vi "U3 Two 32-bit Frequency Measurements.vi"() -> ()   [LabVIEW 2021]
panel:
  out "Frequency (FIO5)":dbl format="%.2f"
  out "Period (FIO5)":dbl format="%.6f"
  out "Iteration":i32
  out "Frequency (FIO4)":dbl format="%.2f"
  out "Period (FIO4)":dbl format="%.6f"
  in  "error in":errorcluster
  in  "Address":string="1"
  in  "FirstFound":bool=TRUE
  in  "stop":bool
  out "Counter1 Diff (FIO6)":u32
  out "error out":errorcluster
  out "Error Message":string
  # "Each iteration, this VI measures the frequency on FIO4 and FIO5 using timer mode 2 (32-bit\nperiod measurement).  Also reads the count on FIO6 and\ndisplays the difference from the previous iteration, with the idea that the same signal can\nbe connected to FIO4/FIO5 and FIO6 for comparison of period timing\nversus pulse counting."
  # "seconds"
  # "seconds"
  # "This VI passes a timer\nbase clock constant that\nis valid for hardware V1.21.\nFor hardware V1.20 change\nLJ_tc48MHZ_DIV to LJ_tc24MHZ_DIV."
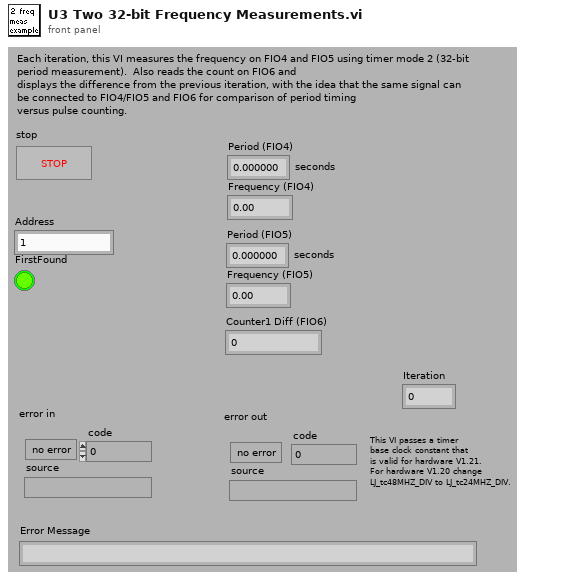
[diagram p1: front panel]
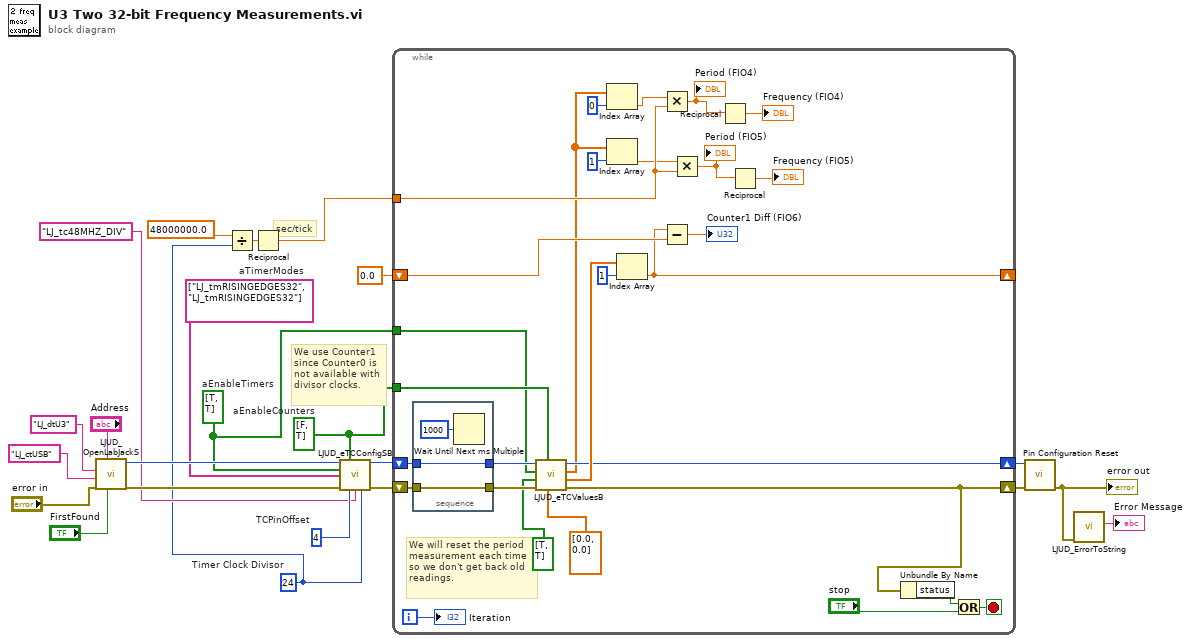
[diagram p0: block diagram]
diagram:
  w8 = 4  # TCPinOffset
  w5 = bool[] [FALSE, TRUE]  # aEnableCounters
  w4 = bool[] [TRUE, TRUE]  # aEnableTimers
  w6 = 24  # Timer Clock Divisor
  w9 = string[] ["LJ_tmRISINGEDGES32", "LJ_tmRISINGEDGES32"]  # aTimerModes
  # "We use Counter1\nsince Counter0 is\nnot available with\ndivisor clocks."
  # "sec/tick"
  n1 = call "LJUD_OpenLabJackS.vi"("FirstFound"="FirstFound", "Address"="Address", "error in"="error in", "ConnectionType"="LJ_ctUSB", "DeviceType"="LJ_dtU3") -> ("error out"=w13:errorcluster, "Handle"=w12:i32)  [unwired: 4 in, 1 out]
  n2 = Divide(x=48000000.0, y=w6) -> (x/y=w18:dbl)
  n3 = Reciprocal(x=w18) -> (1/x=w17:dbl)
  n4 = call "LJUD_eTCConfigSB.vi"("Handle In"=w12, "aEnableCounters"=w5, "aEnableTimers"=w4, "aTimerModes"=w9, "error in"=w13, "TCPinOffset"=w8, "TimerClockBase"="LJ_tc48MHZ_DIV" ("Timer Clock Base"), "TimerClockDivisor"=w6) -> ("Handle Out"=w11:i32, "error out"=w10:errorcluster)  [unwired: 6 in]
  n5 = while {
    tunnel: w4 -> [w25]
    tunnel: w5 -> [w27]
    shift-left: 0.0 ("TimerClockConfig") -> [w40]
    shift-right: [w38] -> _
    tunnel: w17 -> [w33]
    shift-left: w10 -> [w51]
    shift-right: [w31] -> w2
    shift-left: w11 -> [w52]
    shift-right: [w32] -> w3
    i -> [w37]
    stop <- w45 stop-if-true
    # "We will reset the period\nmeasurement each time\nso we don't get back old\nreadings."
    n6 = stacked-sequence {
      tunnel: [w54] -> w48
      tunnel: [w53] -> w47
      tunnel: w52 -> [w54]
      tunnel: w51 -> [w53]
      frame #0 {
        n7 = Wait Until Next ms Multiple(millisecond multiple=u32 1000) -> ()  [unwired: 1 out]
      }
    }
    n8 = call "LJUD_eTCValuesB.vi"("aTimerValues Write"=dbl[] [0.0, 0.0] ("TimerValues"), "aReadCounters"=w27, "error in"=w47, "aUpdateResetTimers"=bool[] [TRUE, TRUE] ("UpdateReset Timers"), "aReadTimers"=w25, "Handle In"=w48) -> ("error out"=w31:errorcluster, "aCounterValues"=w50:dbl[], "aTimerValues Read"=w28:dbl[], "Handle Out"=w32:i32)  [unwired: 2 in]
    n9 = Index Array(array=w28, index=0 ("Index")) -> (element=w34:dbl)
    n10 = Index Array(array=w28, index=1 ("Index")) -> (element=w30:dbl)
    n11 = Index Array(array=w50, index=1 ("Index")) -> (element=w38:dbl)
    n12 = Multiply(x=w34, y=w33) -> (x*y=w42:dbl)
    "Period (FIO4)" <- w42
    n13 = Subtract(x=w38, y=w40) -> (x-y=→"Counter1 Diff (FIO6)":dbl)
    n14 = Multiply(x=w30, y=w33) -> (x*y=w36:dbl)
    "Period (FIO5)" <- w36
    n15 = Reciprocal(x=w42) -> (1/x=→"Frequency (FIO4)":dbl)
    n16 = Reciprocal(x=w36) -> (1/x=→"Frequency (FIO5)":dbl)
    n17 = Unbundle By Name(w31) -> ("status"=w44:bool)
    n18 = Or(x=w44, y="stop") -> (x .or. y?=w45:bool)
    "Iteration" <- w37
  }
  n19 = call "Pin Configuration Reset.vi"("error in"=w2, "Handle In"=w3) -> ("error out"=w1:errorcluster)  [unwired: 8 in, 1 out]
  "error out" <- w1
  n20 = call "LJUD_ErrorToString.vi"("error in"=w1) -> ("String"=→"Error Message":string)  [unwired: 10 in]
